vi "Into Tree Control Items.vi"(10 "Paths Set":set{string}(c389), 11 "Tree Map In":T1) -> (3 "Tree Control Item":T2(array[cluster]))   [LabVIEW 2019, in "Tree Map.lvlib"]
doc: "Helper function for converting the Tree Map elements into Tree Control Items. If you would like to unflatten the data in a different way, modify glyps or change the Tree Control Items array, you can copy and modify the code of this VI or make your changes after or before it runs.\n\n<b>Author:</b> Piotr Kruczkowski <PrimaryKey>\n<b>License:</b> NewBSD\n\nCopyright (c) 2019, National Instruments\nAll rights reserved.\n\nRedistribution and use in source and binary forms, with or without\nmodification, are permitted provided that the following conditions are met:\n1. Redistributions of source code must retain the above copyright\n notice, this list of conditions and the following disclaimer.\n2. Redistributions in binary form must reproduce the above copyright\n notice, this list of conditions and the following disclaimer in the\n documentation and/or other materials provided with the distribution.\n3. Neither the name of National Instruments nor the\n names of its contributors may be used to endorse or promote products\n derived from this software without specific prior written permission.\n\nTHIS SOFTWARE IS PROVIDED BY National Instruments ''AS IS'' AND ANY\nEXPRESS OR IMPLIED WARRANTIES, INCLUDING, BUT NOT LIMITED TO, THE IMPLIED\nWARRANTIES OF MERCHANTABILITY AND FITNESS FOR A PARTICULAR PURPOSE ARE\nDISCLAIMED. IN NO EVENT SHALL National Instruments BE LIABLE FOR ANY\nDIRECT, INDIRECT, INCIDENTAL, SPECIAL, EXEMPLARY, OR CONSEQUENTIAL DAMAGES\n(INCLUDING, BUT NOT LIMITED TO, PROCUREMENT OF SUBSTITUTE GOODS OR SERVICES;\nLOSS OF USE, DATA, OR PROFITS; OR BUSINESS INTERRUPTION) HOWEVER CAUSED AND\nON ANY THEORY OF LIABILITY, WHETHER IN CONTRACT, STRICT LIABILITY, OR TORT\n(INCLUDING NEGLIGENCE OR OTHERWISE) ARISING IN ANY WAY OUT OF THE USE OF THIS\nSOFTWARE, EVEN IF ADVISED OF THE POSSIBILITY OF SUCH DAMAGE."
uses:
  Tree Map.lvlib
  Tree Map Data.ctl
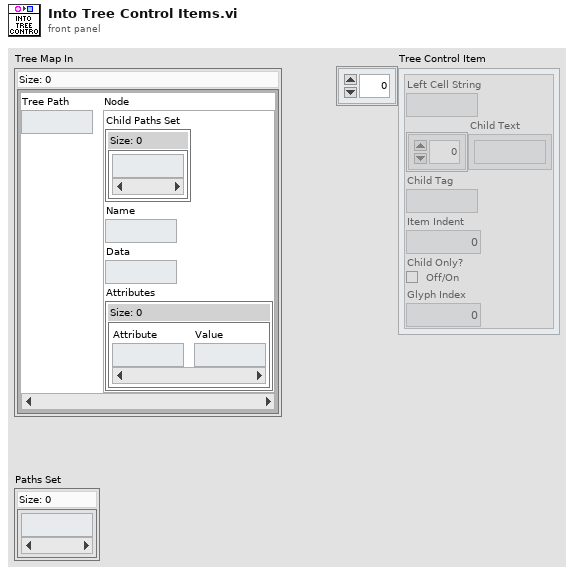
[diagram p1: front panel]
types:
  T1 = typedef "Tree Map.lvlib/Tree Map Data.ctl" = map{string, cluster{"Child Paths Set":set{string}, "Name":string, "Data":string, "Attributes":map{string, string}}}
  T2 = cluster{"Left Cell String":string, "Child Text":string[], "Child Tag":string, "Item Indent":i32, "Child Only?":bool, "Glyph Index":i32}[]
  T3 = cluster{"Left Cell String":string, "Child Text":string[], "Child Tag":string, "Item Indent":i32, "Child Only?":bool, "Glyph Index":i32}
  T4 = cluster{"Child Paths Set":set{string}, "Name":string, "Data":string, "Attributes":map{string, string}}
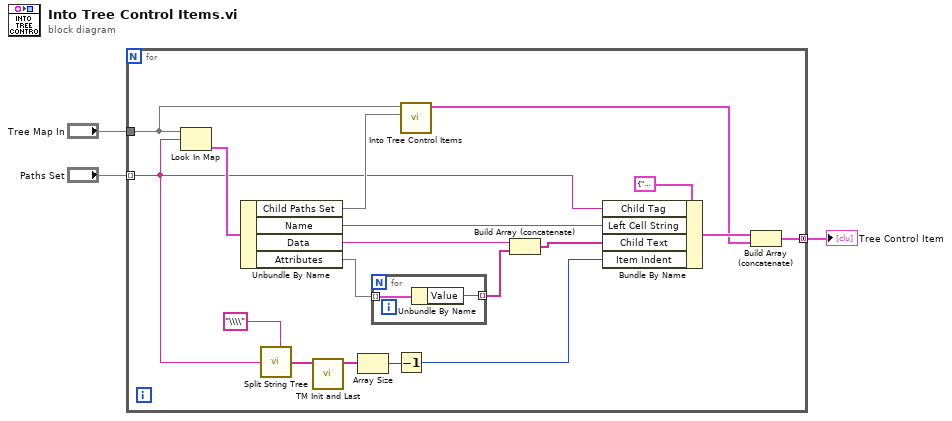
[diagram p0: block diagram]
diagram:
  n1 = for {
    tunnel: "Paths Set" -> [w12] mode=indexing
    tunnel: [w4] -> w1 mode=concatenating
    tunnel: "Tree Map In" -> [w20]
    n2 = Look In Map(map=w20, key=w12) -> (value=w21:T4)  [unwired: 1 in, 1 out]
    n3 = Unbundle By Name(w21) -> ("Child Paths Set"=w19:set{string}, "Name"=w17:string, "Data"=w8:string, "Attributes"=w11:map{string, string})
    n4 = call "Split String Tree.vi"("Split Pattern"="\\\\", "Input String"=w12) -> ("Split String"=w13:string[])  [unwired: 5 in]
    n5 = call "TM Init and Last.vi"("List"=w13) -> ("Init List"=w15:string[])  [unwired: 9 in, 1 out]
    n6 = Array Size(array=w15) -> (size(s)=w16:i32)
    n7 = for {
      tunnel: w11 -> [w23] mode=indexing
      tunnel: [w22] -> w9 mode=indexing
      n8 = Unbundle By Name(w23) -> ("Value"=w22:string)
    }
    n9 = Decrement(x=w16) -> (x-1=w10:i32)
    n10 = call "Into Tree Control Items.vi"("Paths Set"=w19, "Tree Map In"=w20) -> ("Tree Control Item"=w5:T2)  [unwired: 9 in]
    n11 = Build Array (concatenate)(w8, w9) -> (w7:string[])
    n12 = Bundle By Name(cluster=T3 {"Left Cell String"="", "Child Text"=[], "Child Tag"="", "Item Indent"=0, "Child Only?"=FALSE, "Glyph Index"=0} ("Item"), "Child Tag"=w12, "Left Cell String"=w17, "Child Text"=w7, "Item Indent"=w10) -> (w6:T3)
    n13 = Build Array (concatenate)(w6, w5) -> (w4:T2)
  }
  "Tree Control Item" <- w1
